vi "Global_Cal STD.vi"() -> ()   [LabVIEW 2020]
panel:
  in  "E/M Select":string
  in  "STD List":string[][](array[string])
  in  "Cal STD":string[][](array[string])
  # "DSEQ, ISID, STDNAM, C1_VAL, C2_VAL, C3_VAL, C4_VAL, C5_VAL, C6_VAL, C7_VAL, C8_VAL, C9_VAL, C10_VAL, NOMN, STD, MEAS, UNIT_1, CORR, UNIT_2, UNC_1, UNC_2, UNIT_3, K, REMARK\nCOEF_1, COEF_2, COEF_3, COEF_4, COEF_5, COEF_6, COEF_7, COEF_8, COEF_9, COEF_10, CALDATE"
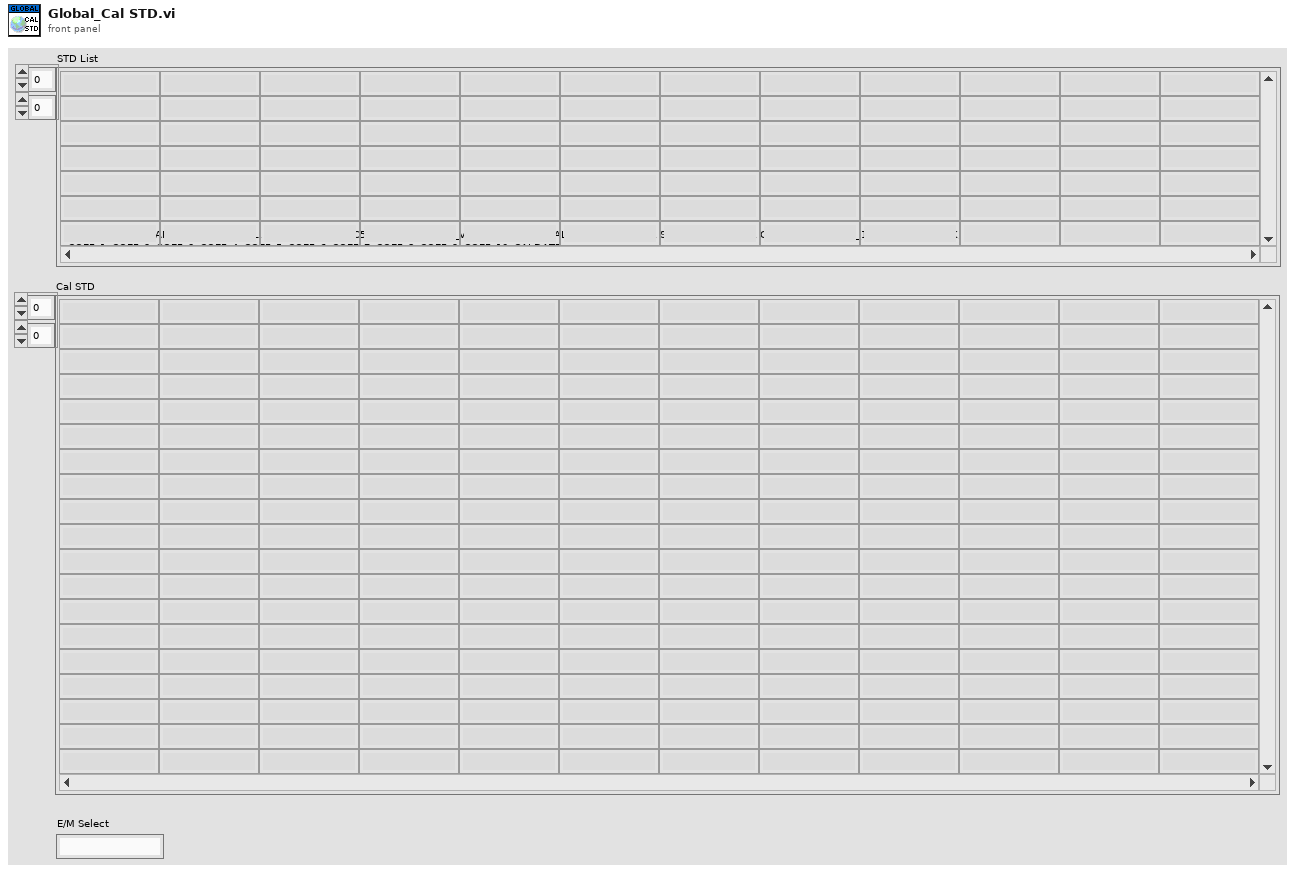
[diagram p1: front panel]
diagram:
